vi "模版模式DEMO.vi"() -> ()   [LabVIEW 2013]
uses:
  Adlink_class/Adlink.lvclass
  Advantech_class/Advantech.lvclass
  AD_class/AD.lvclass
  <vilib>/addons/_AddQ/G#Object/G#Object.lvclass
panel:
  out "# of objects killed":i32
  in  "停止":bool
  out "温度与力":dbl[](array[numeric])
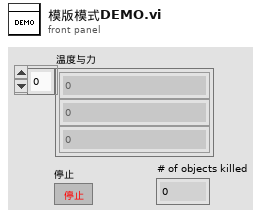
[diagram p1: front panel]
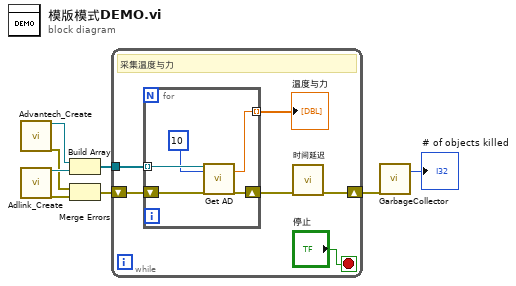
[diagram p0: block diagram]
diagram:
  n1 = call "Advantech_Create.vi"() -> ("reference out"=w8:refnum<class "Advantech.lvclass">, "error out"=w5:errorcluster)  [unwired: 18 in]
  n2 = call "Adlink_Create.vi"() -> ("reference out"=w7:refnum<class "Adlink.lvclass">, "error out"=w4:errorcluster)  [unwired: 18 in]
  n3 = Build Array(w8, w7) -> (w6:refnum<class "AD.lvclass">[])
  n4 = Merge Errors(w5, w4) -> (w3:errorcluster)
  n5 = while {
    tunnel: w6 -> [w14]
    shift-right: [w9] -> w2
    shift-left: w3 -> [w11]
    stop <- "停止" stop-if-true
    # "采集温度与力"
    n6 = for {
      tunnel: w14 -> [w19] mode=indexing
      tunnel: [w17] -> w13 mode=indexing
      shift-right: [w15] -> w10
      shift-left: w11 -> [w16]
      n7 = call "Get AD.vi"("reference in"=w19, "Count"=10, "error in (no error)"=w16) -> ("Value"=w17:dbl, "error out"=w15:errorcluster)  [unwired: 14 in, 1 out]
    }
    "温度与力" <- w13
    n8 = call "时间延迟"("error in (no error)"=w10) -> ("error out"=w9:errorcluster)  [unwired: 10 in]
  }
  n9 = call <vilib>:"GarbageCollector.vi"("error in (no error)"=w2) -> ("# of objects killed"=→"# of objects killed":i32)  [unwired: 16 in, 2 out]
